vi "Agilent SNA Set Format.vi"(6 "Channel":i8=1 min=1 max=99 step=1, 7 "Agilent SNA & SWP":T1, 8 "error in (no error)":errorcluster, 10 "Display Format":T3, 11 "VISA Resource Names":T2) -> (0 "error out":errorcluster, 3 "dup VISA Resource Names":T2)   [LabVIEW 2011]
doc: "This VI for the HP 8753B is used to read the meausurement format.\n\n0 log magnitude\n1 phase\n2 delay\n3 Smith chart\n4 polar\n5 linear magnitude\n6 standing wave ratio\n7 real\n8 imaginary"
uses:
  SNA Measurement Format.ctl
  TypeDefs/Agilent SNA VISA.ctl
  TypeDefs/Agilent SNA Instrument Info.ctl
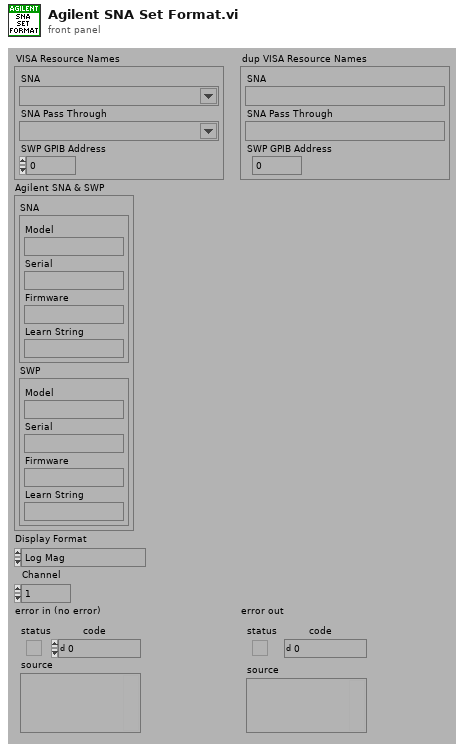
[diagram p1: front panel]
types:
  T1 = typedef "Agilent SNA Instrument Info.ctl" = cluster{"SNA":cluster{"Model":string, "Serial":string, "Firmware":string, "Learn String":string}, "SWP":cluster{"Model":string, "Serial":string, "Firmware":string, "Learn String":string}}
  T2 = typedef "Agilent SNA VISA.ctl" = cluster{"SNA":refnum<visa-resource-name>, "SNA Pass Through":refnum<visa-resource-name>, "SWP GPIB Address":i32}
  T3 = typedef "SNA Measurement Format.ctl" = enum32{"Log Mag", "Normalized Log Mag", "SWR", "Linear Mag", "Power Out"}
  T4 = typedef "Agilent SNA Model.ctl" = enum16{"Not Supported", "8757X"}
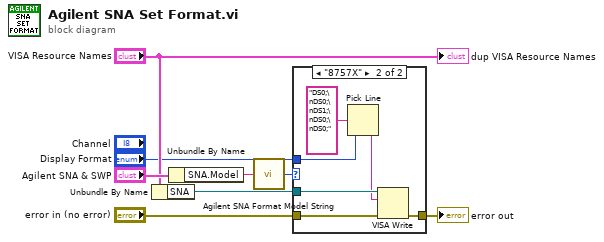
[diagram p0: block diagram]
diagram:
  n1 = Unbundle By Name("VISA Resource Names") -> ("SNA"=w2:refnum<visa-resource-name>)
  n2 = Unbundle By Name("Agilent SNA & SWP") -> ("SNA.Model"=w4:string)
  n3 = call "Agilent SNA Format Model String.vi"("Model String"=w4) -> ("Model"=w6:T4)
  n4 = case shown="\"8757X\"" w6 {
    tunnel: "error in (no error)" -> [w9 w15]
    tunnel: [w9 w14] -> w7
    tunnel: w2 -> [_ w13]
    tunnel: "Display Format" -> [_ w11]
    frame "Not Supported" {
    }
    frame "8757X" {
      n5 = Pick Line(multi-line string="DS0;\nDS0;\nDS1;\nDS0;\nDS0;", line index=w11) -> (output string=w12:string)  [unwired: 1 out]
      n6 = VISA Write(VISA resource name=w13, write buffer=w12, error in (no error)=w15) -> (error out=w14:errorcluster)  [unwired: 2 out]
    }
  }
  "error out" <- w7
  "dup VISA Resource Names" <- "VISA Resource Names"
